vi "Set Sweep Frequency.vi"(7 "Sweep Frequency":T1, 8 "error in (no error)":errorcluster, 9 "frequency":dbl[unit], 10 "Channel (0: Channel 1)":T2 items=["Channel 1", "Channel 2"], 11 "VISA resource name":refnum<visa-resource-name>) -> (0 "error out":errorcluster, 3 "VISA resource name out":refnum<visa-resource-name>)   [LabVIEW 2023, in "Tektronix AFG 3000 Series.lvlib"]
doc: "Sets the specified sweep frequency (center, span, start, or stop) of a Tektronix AFG 3000 series function generator. Used in sweep mode. <B>Note:</B> if you change the output waveform, this frequency may change, since the range of frequencies available will be different."
uses:
  Tektronix AFG 3000 Series.lvlib
  controls.llb/Channel.ctl
  controls.llb/Sweep Frequency.ctl
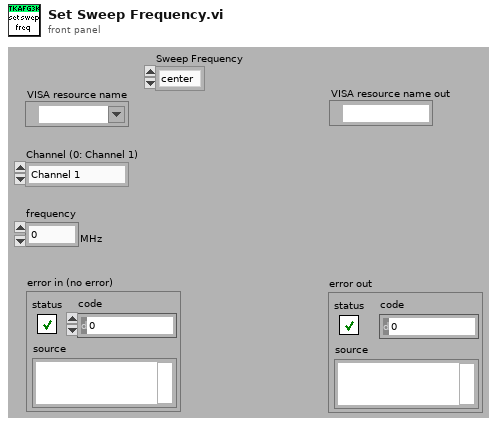
[diagram p1: front panel]
types:
  T1 = typedef "Sweep Frequency.ctl" = enum16{"center", "span", "start", "stop"}
  T2 = typedef "Channel.ctl" = u16
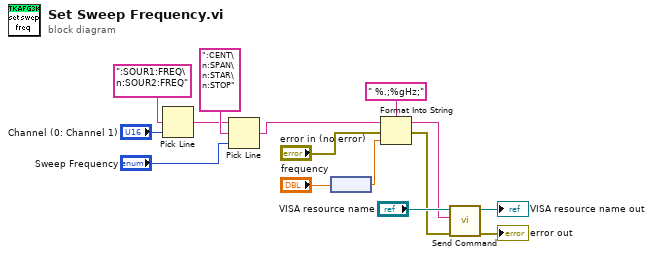
[diagram p0: block diagram]
diagram:
  n1 = Pick Line(multi-line string=":SOUR1:FREQ\n:SOUR2:FREQ", line index="Channel (0: Channel 1)") -> (output string=w2:string)  [unwired: 1 out]
  n2 = Pick Line(string ("")=w2, multi-line string=":CENT\n:SPAN\n:STAR\n:STOP" ("format string"), line index="Sweep Frequency") -> (output string=w1:string)
  n3 = node("frequency") -> (w10:dbl)
  n4 = Format Into String(format string=" %.;%gHz;", initial string=w1, error in="error in (no error)", w10) -> (resulting string=w9:string, error out=w7:errorcluster)
  n5 = call "Send Command.vi"("error in (no error)"=w7, "write buffer"=w9, "VISA resource name"="VISA resource name") -> ("error out"=→"error out":errorcluster, "VISA resource name out"=→"VISA resource name out":refnum<visa-resource-name>)  [unwired: 7 out]
